vi "My SIM PID Derivative Gain.vi"(2 "Derivative Gain":dbl, 7 "Error":dbl, 13 "High Frequency [s] (Tf)":dbl=1.0) -> (8 "output":dbl)   [LabVIEW 2012]
uses:
  <vilib>/Simulation/Implementation/Shared/SIMSCR Execution Mode.ctl
  <vilib>/Simulation/Scripting/Companion Diagram/SimConfigNode/SimParams.ctl
  <vilib>/Simulation/Scripting/Companion Diagram/SimConfigNode/_simSolvers.ctl
  <vilib>/Simulation/Param Hierarchy/Typedefs/SIMPH Param Control Actions.ctl
  <vilib>/Simulation/Implementation/Shared/NILVSim_ParamChanged.vi
  <vilib>/Simulation/SignalArithmetic/Implementation/NILVSim Gain.llb/SIM Gain (scalar).vi
  <vilib>/Simulation/Implementation/Shared/SIM Is Init or Final Stage.vi
  <vilib>/Simulation/ContinuousLinear/Implementation/NILVSim Transfer Function Direct.llb/SIM Transfer Function Direct (SISO).vi
  <vilib>/Simulation/Implementation/Shared/NILVSim_Manager.vi
  <vilib>/Simulation/Implementation/Shared/NILVSim_FinalizeModel.vi
  <vilib>/Simulation/Implementation/Shared/SIM Unbundle Sim Info.vi
  <vilib>/Utility/error.llb/Clear Errors.vi
  <vilib>/Simulation/Implementation/Shared/NILVSim_GetModelError.vi
  <vilib>/Simulation/Implementation/Shared/SIM SimErrorHandler.vi
  <vilib>/Simulation/Implementation/Shared/SIM Bundle Sim Info.vi
  <vilib>/Simulation/Implementation/Shared/SIMSH Read Queue.vi
  <vilib>/Simulation/Implementation/Shared/NILVSim_Initialize.vi
  <vilib>/Simulation/Utility/Implementation/NILVSim Get Time and IsAcceptedStep.vi
  <vilib>/Simulation/Scripting/Companion Diagram/SimConfigNode/SimDog.xnode
  <vilib>/Simulation/Implementation/XNodeFramework/SimXNode/SimX.xnode
  <vilib>/Simulation/Implementation/Shared/NI_SIM_Implementation.lvlib
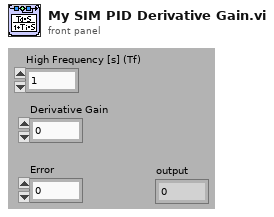
[diagram p1: front panel]
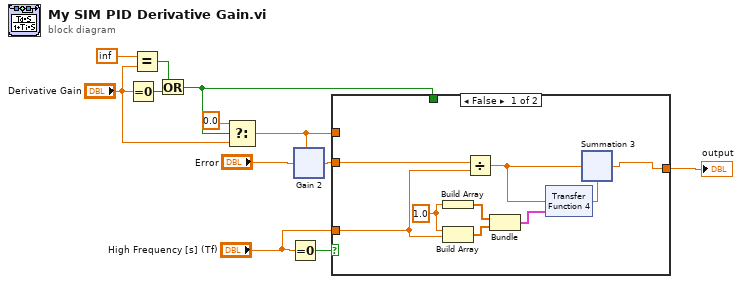
[diagram p0: block diagram]
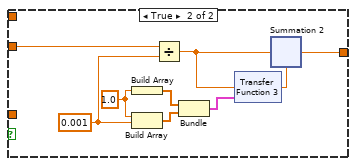
[diagram p2: hidden frame]
diagram:
  n1 = Equal To 0?(x="Derivative Gain") -> (x = 0?=w9:bool)
  n2 = Equal?(x=inf ("Constant 2"), y="Derivative Gain") -> (x = y?=w7:bool)
  n3 = Or(x=w7, y=w9) -> (x .or. y?=w4:bool)
  n4 = Select ("Select 2")(t=0.0 ("t 3"), s=w4, f="Derivative Gain") -> (s? t:f=w5:dbl)
  n5 = Equal To 0? ("Equal To 0? 2")(x="High Frequency [s] (Tf)") -> (x = 0?=w1:bool)
  n6 = xnode ("Gain 2")("gain"=w5, "input"="Error") -> ("output"=w2:dbl)  [unwired: 2 in]
  n7 = case "Case Structure 2" shown="False" w1 {
    tunnel: w2 -> [w21 w39]
    tunnel: [w20 w40] -> w11
    tunnel: "High Frequency [s] (Tf)" -> [w19 _]
    tunnel: w4 -> [_ _]
    tunnel: w5 -> [_ _]
    frame False {
      w14 = 1.0 ("element 6")
      n8 = Build Array ("Build Array 7")(w14) -> (w16:dbl[])
      n9 = Build Array ("Build Array 8")(w14, w19) -> (w15:dbl[])
      n10 = Divide ("Divide 2")(x=w21, y=w19) -> (x/y=w13:dbl)
      n11 = Bundle ("Bundle 5")(w16, w15) -> (w17:cluster{dbl[], dbl[]})  [unwired: 1 in]
      n12 = xnode ("Transfer Function 4")("input u(k)"=w13, "Transfer Function"=w17) -> ("output y(k)"=w18:dbl)  [unwired: 3 in, 1 out]
      n13 = xnode ("Summation 3")("Operand1"=w13, "Operand2"=w18) -> ("Result"=w20:dbl)
    }
    frame True {
      w32 = 0.001 ("y 2")
      w34 = 1.0 ("element 5")
      n14 = Build Array ("Build Array 5")(w34) -> (w36:dbl[])
      n15 = Build Array ("Build Array 6")(w34, w32) -> (w35:dbl[])
      n16 = Divide(x=w39, y=w32) -> (x/y=w33:dbl)
      n17 = Bundle ("Bundle 4")(w36, w35) -> (w37:cluster{dbl[], dbl[]})  [unwired: 1 in]
      n18 = xnode ("Transfer Function 3")("input u(k)"=w33, "Transfer Function"=w37) -> ("output y(k)"=w38:dbl)  [unwired: 3 in, 1 out]
      n19 = xnode ("Summation 2")("Operand1"=w33, "Operand2"=w38) -> ("Result"=w40:dbl)
    }
  }
  "output" <- w11
